vi "Servo_Button2.vi"() -> ()   [LabVIEW 2018]
uses:
  <vilib>/rvi/Emulation/niFpgaGetClockAttributes.vi
  <vilib>/rvi/Emulation/niFpgaSctlEmulationGetInTimedLoop.vi
  <vilib>/rvi/Emulation/niFpgaEmulationReportErrorSimple.vi
  <vilib>/rvi/eio/common/nirviEmuTemplateMethod_errors.vi
  <vilib>/rvi/Emulation/niFpgaCriticalErrorInLSC.vi
  <vilib>/eio/EIONode/EIONode.xnode
panel:
  in  "Stop":bool
  out "Degree":u32
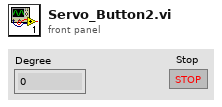
[diagram p1: front panel]
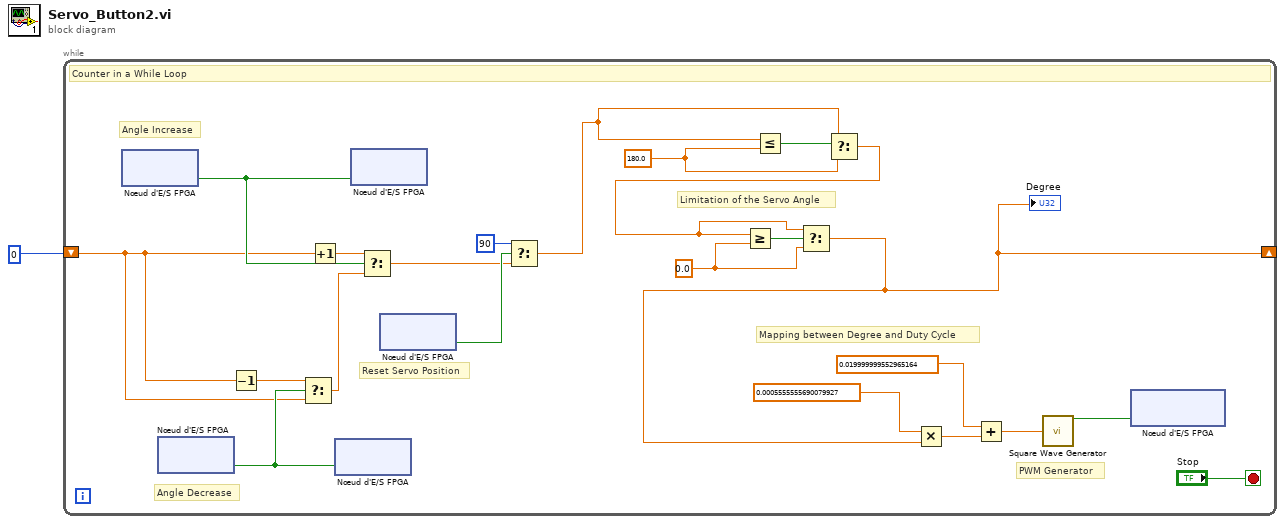
[diagram p0: block diagram]
diagram:
  n1 = while "Timed Loop" {
    shift-right: [w4] -> _
    shift-left: u32 0 -> [w7]
    stop <- "Stop" stop-if-true
    w3 = sgl 0.0
    w6 = sgl 180.0
    # "PWM Generator"
    # "Mapping between Degree and Duty Cycle"
    # "Limitation of the Servo Angle"
    # "Angle Decrease"
    # "Angle Increase"
    # "Reset Servo Position"
    # "Counter in a While Loop"
    n2 = xnode "Nœud d'E/S FPGA"() -> ("BTN1"=w10:bool)  [unwired: 1 in, 1 out]
    n3 = xnode "Nœud d'E/S FPGA"() -> ("BTN2"=w9:bool)  [unwired: 1 in, 1 out]
    n4 = Decrement(x=w7) -> (x-1=w8:sgl)
    n5 = Select(t=w8, s=w9, f=w7) -> (s? t:f=w13:sgl)
    n6 = Increment(x=w7) -> (x+1=w22:sgl)
    n7 = xnode "Nœud d'E/S FPGA"("LED2"=w9) -> ()  [unwired: 1 in, 1 out]
    n8 = xnode "Nœud d'E/S FPGA"("LED1"=w10) -> ()  [unwired: 1 in, 1 out]
    n9 = Select(t=w22, s=w10, f=w13) -> (s? t:f=w14:sgl)
    n10 = xnode "Nœud d'E/S FPGA"() -> ("BTN0"=w21:bool)  [unwired: 1 in, 1 out]
    n11 = Select(t=u32 90, s=w21, f=w14) -> (s? t:f=w11:sgl)
    n12 = Less Or Equal?(x=w11, y=w6) -> (x <= y?=w12:bool)
    n13 = Select(t=w11, s=w12, f=w6) -> (s? t:f=w2:sgl)
    n14 = Greater Or Equal?(x=w2, y=w3) -> (x >= y?=w5:bool)
    n15 = Select(t=w2, s=w5, f=w3) -> (s? t:f=w4:sgl)
    "Degree" <- w4
    n16 = Multiply(x=sgl 0.00055555557, y=w4) -> (x*y=w19:sgl)
    n17 = Add(x=sgl 0.02, y=w19) -> (x+y=w18:sgl)
    n18 = call "Square Wave Generator"("duty cycle (periods)"=w18) -> ("square wave out"=w17:bool)  [unwired: 14 in]
    n19 = xnode "Nœud d'E/S FPGA"("BB3_DIO0"=w17) -> ()  [unwired: 1 in, 1 out]
  }
